vi "Run.vi"(8 "error in (no error)":errorcluster, 11 "fpMgr in":refnum<class "VIProviderShellHelper.lvclass">) -> (0 "error out":errorcluster, 3 "fpMgr out":refnum<class "VIProviderShellHelper.lvclass">)   [LabVIEW 2019, in "LabVIEW-VIProviderShell.lvlib" / "VIProviderShellHelper.lvclass"]
uses:
  VIProviderShellHelper.lvclass
  VIProviderShellHelper.lvclass/VIProviderShellHelper.ctl
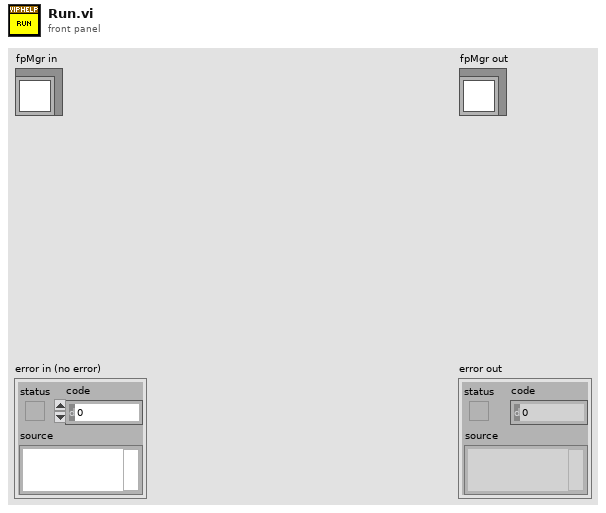
[diagram p1: front panel]
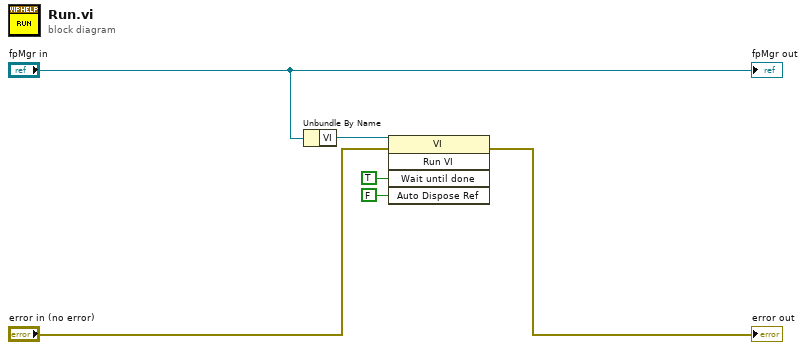
[diagram p0: block diagram]
diagram:
  n1 = Unbundle By Name("fpMgr in") -> ("VI"=w5:refnum<vi>)
  n2 = invoke class="VI" method="Run VI"(reference=w5, error in="error in (no error)", "Wait until done"=TRUE ("Wait Until Done"), "Auto Dispose Ref"=FALSE ("Auto Dispose Reference")) -> (error out=→"error out":errorcluster)  [unwired: 1 in, 4 out]
  "fpMgr out" <- "fpMgr in"
